vi "电流对称性.vi"(9 "索引":i32, 10 "定点":dbl, 11 "XY图":cluster{dbl[], dbl[]}[](graph)) -> (3 "对称性":dbl)   [LabVIEW 2020]
uses:
  <vilib>/Analysis/NI_AAL_Geometry.lvlib
panel:
  out "XY图 2":cluster{dbl[], dbl[]}[](graph)
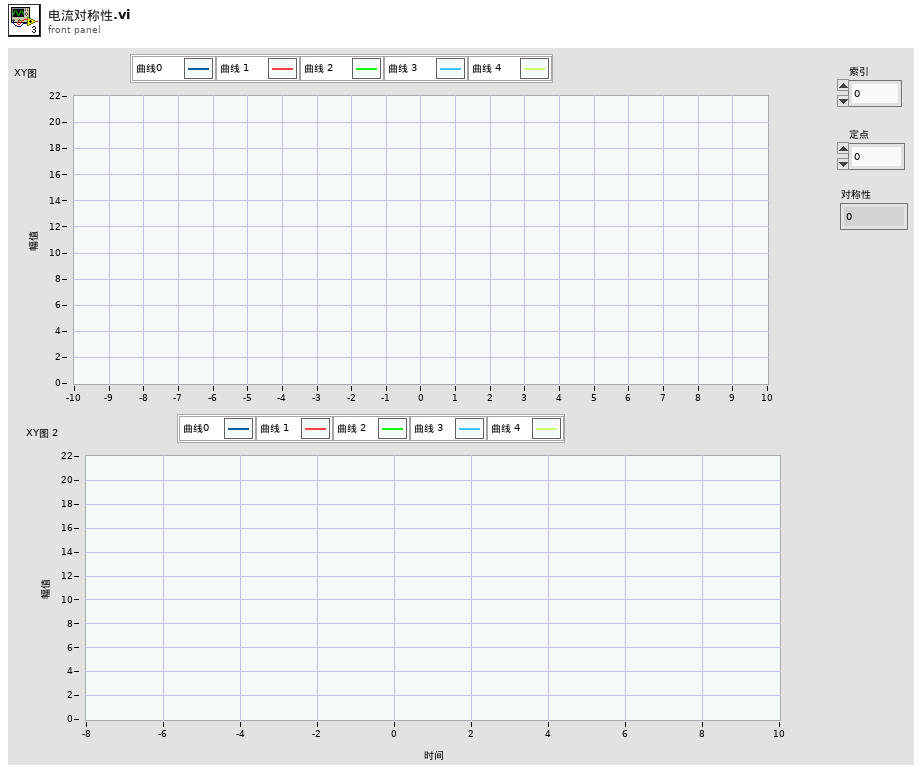
[diagram p1: front panel]
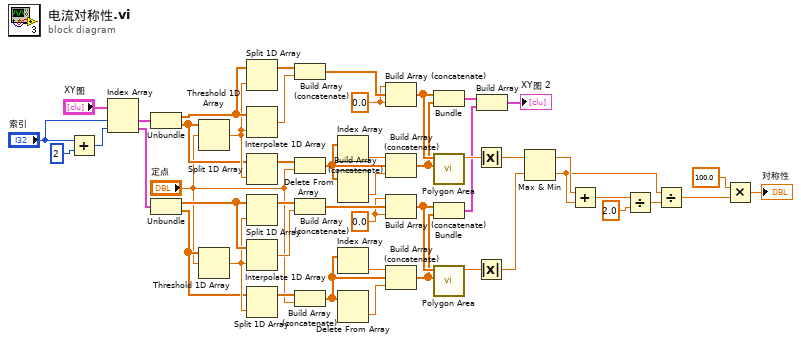
[diagram p0: block diagram]
diagram:
  w33 = 0.0
  w32 = 0.0
  n1 = Add(x="索引", y=2) -> (x+y=w21:i32)
  n2 = Index Array(array="XY图", index #1="索引", index #2=w21) -> (element #1=w35:cluster{dbl[], dbl[]}, element #2=w23:cluster{dbl[], dbl[]})
  n3 = Unbundle(w35) -> (w34:dbl[], w3:dbl[])
  n4 = Unbundle(w23) -> (w19:dbl[], w2:dbl[])
  n5 = Threshold 1D Array(2:"定点", 3:w3) -> (0:w14:dbl)  [unwired: 1 in]
  n6 = Threshold 1D Array(2:"定点", 3:w2) -> (0:w12:dbl)  [unwired: 1 in]
  n7 = Split 1D Array(array=w34, index=w14) -> (first subarray=w18:dbl[])  [unwired: 1 out]
  n8 = Interpolate 1D Array(1:w14, 2:w34) -> (0:w13:dbl)
  n9 = Split 1D Array(array=w3, index=w14) -> (first subarray=w17:dbl[])  [unwired: 1 out]
  n10 = Split 1D Array(array=w19, index=w12) -> (first subarray=w15:dbl[])  [unwired: 1 out]
  n11 = Interpolate 1D Array(1:w12, 2:w19) -> (0:w11:dbl)
  n12 = Split 1D Array(array=w2, index=w12) -> (first subarray=w16:dbl[])  [unwired: 1 out]
  n13 = Build Array (concatenate)(w18, w13) -> (w38:dbl[])
  n14 = Build Array (concatenate)(w17, "定点") -> (w40:dbl[])
  n15 = Build Array (concatenate)(w15, w11) -> (w45:dbl[])
  n16 = Build Array (concatenate)(w16, "定点") -> (w44:dbl[])
  n17 = Index Array(array=w40) -> (element=w39:dbl)  [unwired: 1 in]
  n18 = Delete From Array(array=w40) -> (deleted portion=w41:dbl)  [unwired: 2 in, 1 out]
  n19 = Index Array(array=w44) -> (element=w43:dbl)  [unwired: 1 in]
  n20 = Delete From Array(array=w44) -> (deleted portion=w42:dbl)  [unwired: 2 in, 1 out]
  n21 = Build Array (concatenate)(w32, w38, w32) -> (w10:dbl[])
  n22 = Build Array (concatenate)(w39, w40, w41) -> (w9:dbl[])
  n23 = Build Array (concatenate)(w33, w45, w33) -> (w8:dbl[])
  n24 = Build Array (concatenate)(w43, w44, w42) -> (w7:dbl[])
  n25 = Bundle(w10, w9) -> (w6:cluster{dbl[], dbl[]})  [unwired: 1 in]
  n26 = call <vilib>:"Polygon Area.vi"("Y"=w9, "X"=w10) -> ("signed area"=w37:dbl)  [unwired: 8 in, 1 out]
  n27 = Bundle(w8, w7) -> (w5:cluster{dbl[], dbl[]})  [unwired: 1 in]
  n28 = call <vilib>:"Polygon Area.vi"("Y"=w7, "X"=w8) -> ("signed area"=w36:dbl)  [unwired: 8 in, 1 out]
  n29 = Absolute Value(x=w37) -> (abs(x)=w31:dbl)
  n30 = Absolute Value(x=w36) -> (abs(x)=w30:dbl)
  n31 = Build Array(w6, w5) -> (→"XY图 2":cluster{dbl[], dbl[]}[])
  n32 = Max & Min(x=w31, y=w30) -> (max(x,y)=w29:dbl, min(x,y)=w26:dbl)
  n33 = Add(x=w29, y=w26) -> (x+y=w28:dbl)
  n34 = Divide(x=w28, y=2.0) -> (x/y=w25:dbl)
  n35 = Divide(x=w26, y=w25) -> (x/y=w24:dbl)
  n36 = Multiply(x=100.0, y=w24) -> (x*y=→"对称性":dbl)
